vi "Sample Changer tester.vi"() -> ()   [LabVIEW 2016]
uses:
  Tester-states.ctl
  <vilib>/Analysis/NI_AALBase.lvlib
panel:
  out "Rotation Duration":u32(graph)
  out "Rotation Duration Histogram":T1(graph)
  out "End Time":timestamp
  out "Start Time":timestamp
  out "Error Histogram":T1(graph)
  out "Success rate":dbl
  in  "Trials":i32=5
  out "Sample Number":cluster{"UInt8":u8, "UInt8":u8}(graph)
  in  "Rotate minimum time":u32=5000
  out "Position error (encoder steps)":i32(graph)
  out "Encoder data":cluster{"Int32":i32, "Int32":i32}(graph)={"Int32"=515, "Int32"=0}
  out "Encoder Destination":i32
  out "Encoder Position":i32
  out "Current Sample":u8
  out "Loop Counter":i32
  in  "Encoder Radius":dbl=2.0
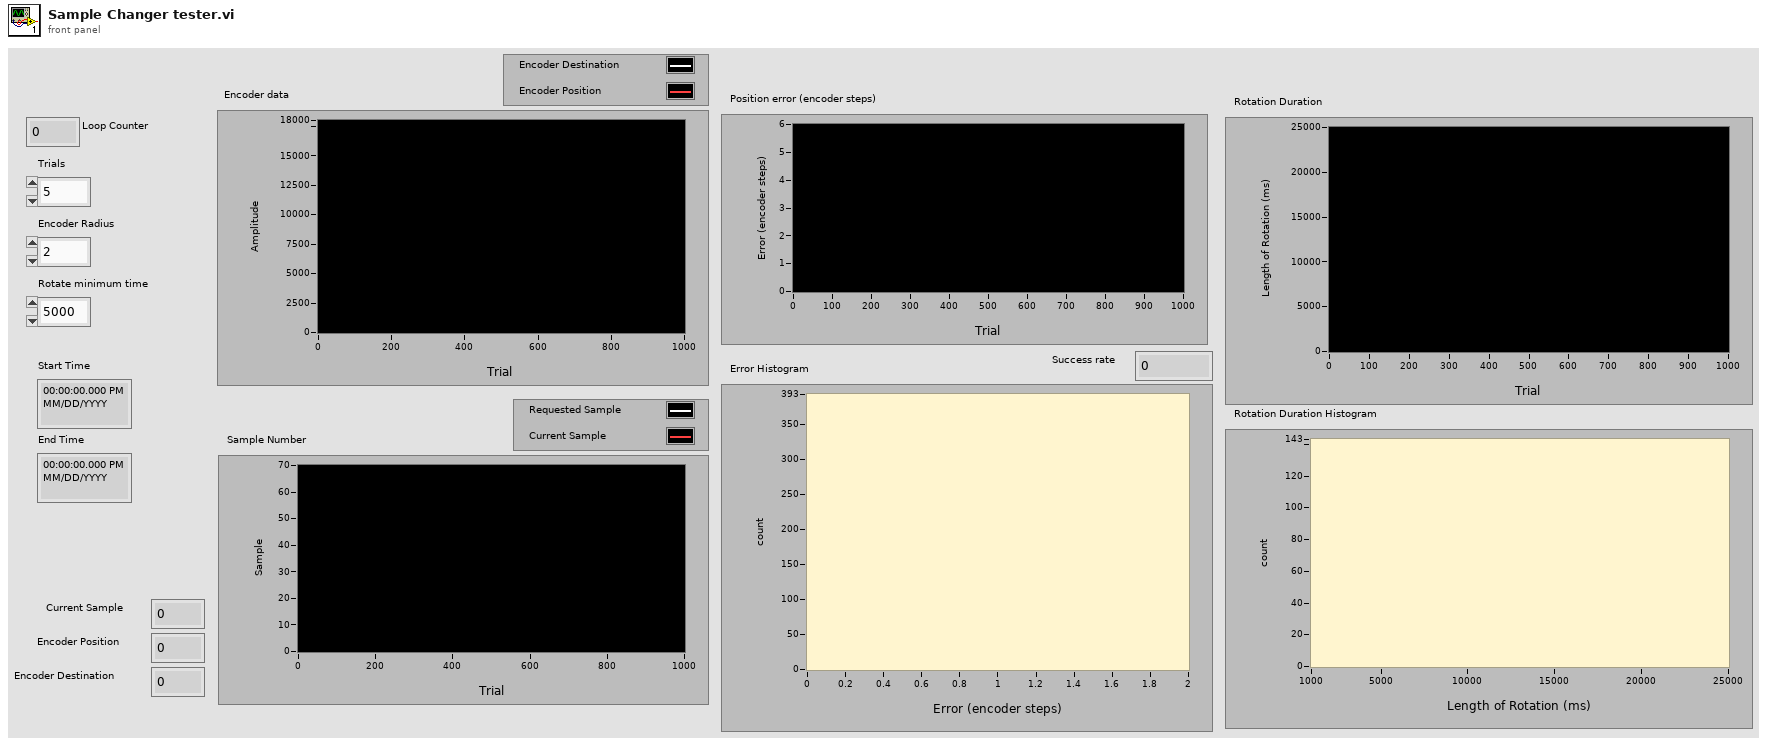
[diagram p1: front panel]
types:
  T1 = cluster{"X Values":dbl[], "Histogram: h(x)":i32[]}
  T2 = typedef "Tester-states.ctl" = enum16{"wait", "start trial", "get trial data", "test complete"}
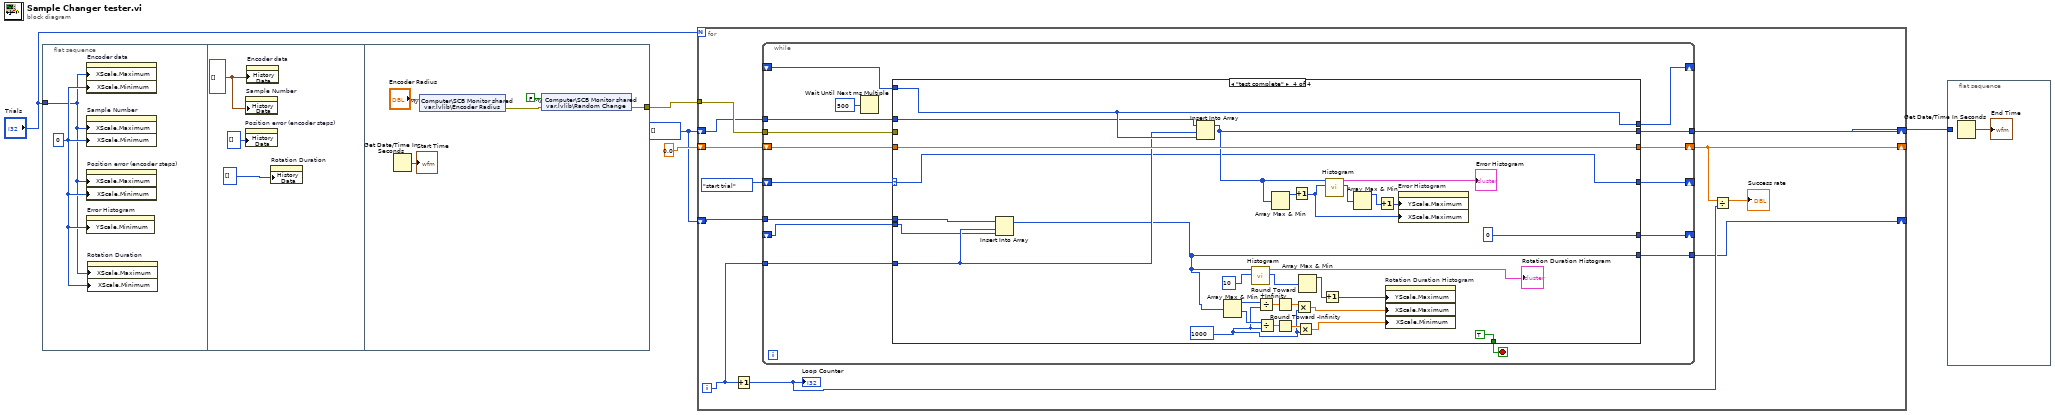
[diagram p0: block diagram]
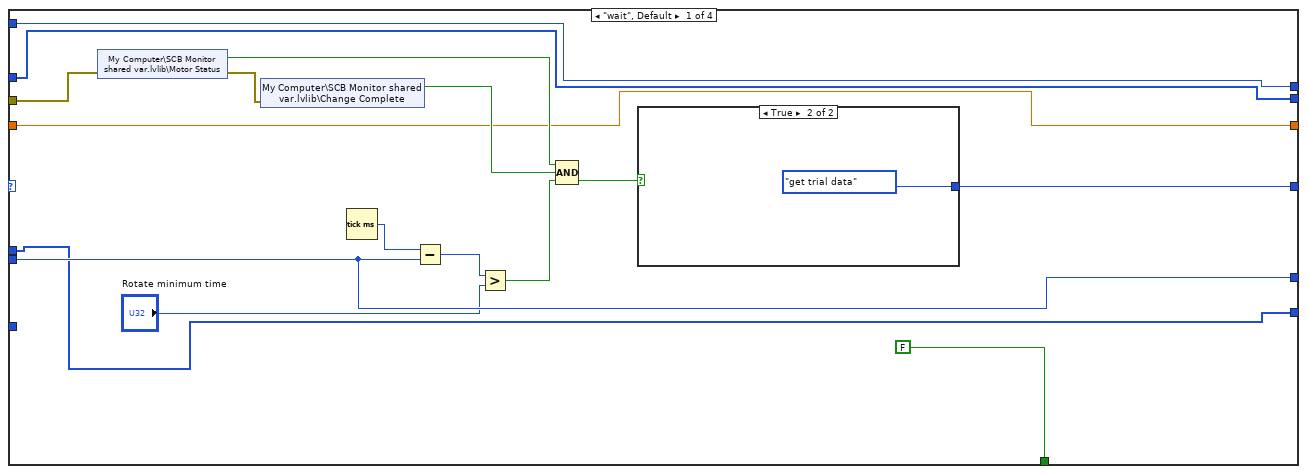
[diagram p2: hidden frame]
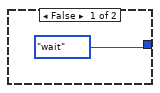
[diagram p3: hidden frame]
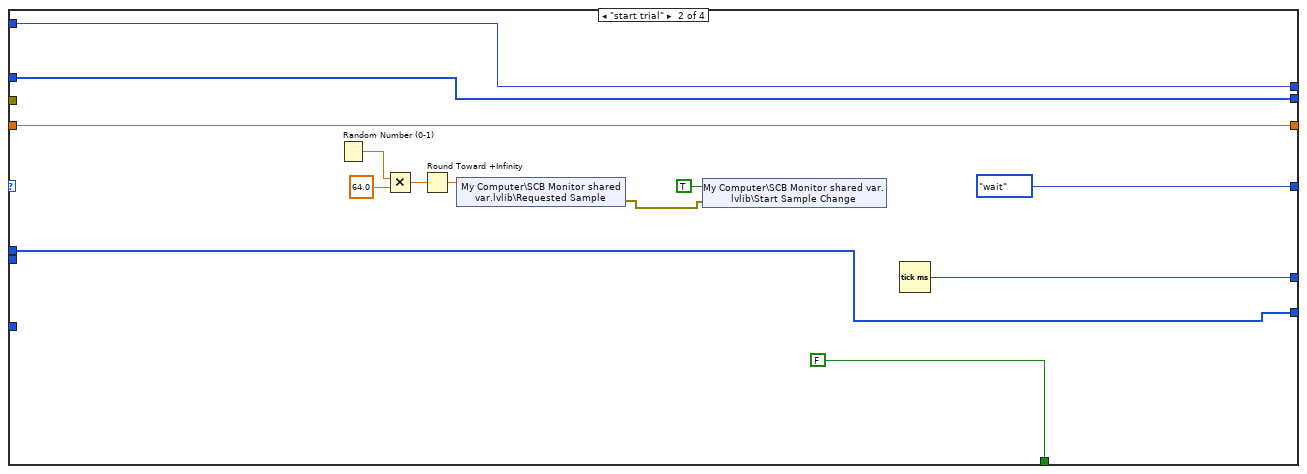
[diagram p4: hidden frame]
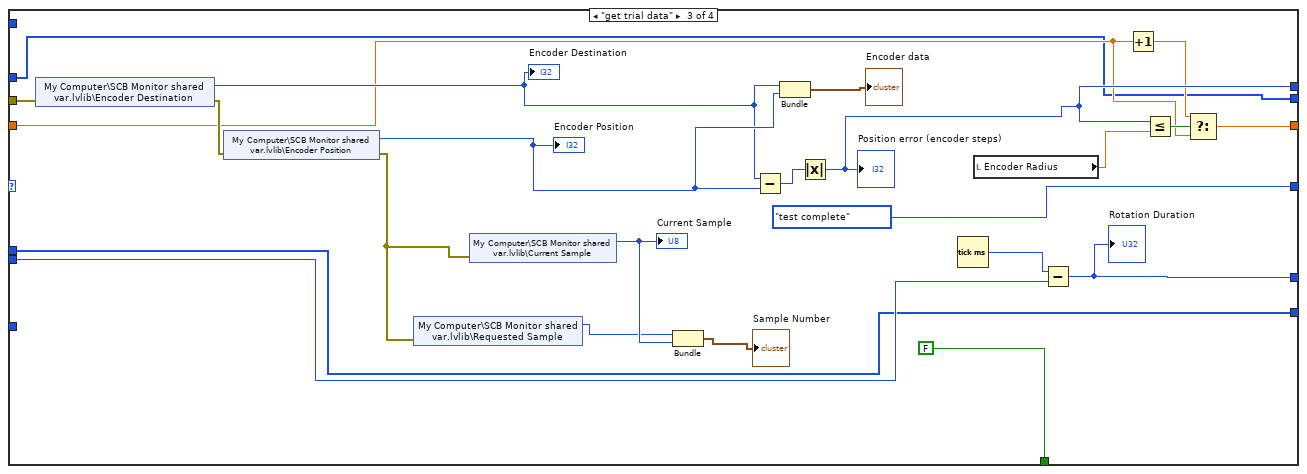
[diagram p5: hidden frame]
diagram:
  w1 = i32[] []
  n1 = flat-sequence {
    tunnel: "Trials" -> [w6]
    tunnel: [w12] -> w5
    frame #0 {
      w7 = 0 ("Trials 2")
      n2 = property on="Encoder data" class="WFChart (strict)"("XScale.Maximum"=w6, "XScale.Minimum"=w7) -> ()  [unwired: 2 in, 2 out]
      n3 = property on="Sample Number" class="WFChart (strict)"("XScale.Maximum"=w6, "XScale.Minimum"=w7) -> ()  [unwired: 2 in, 2 out]
      n4 = property on="Position error (encoder steps)" class="WFChart (strict)"("XScale.Maximum"=w6, "XScale.Minimum"=w7) -> ()  [unwired: 2 in, 2 out]
      n5 = property on="Error Histogram" class="XYGraph (strict)"("YScale.Minimum"=w7) -> ()  [unwired: 2 in, 2 out]
      n6 = property on="Rotation Duration" class="WFChart (strict)"("XScale.Maximum"=w6, "XScale.Minimum"=w7) -> ()  [unwired: 2 in, 2 out]
    }
    frame #1 {
      w9 = cluster{"Int32":i32, "Int32":i32}[] [] ("History Data")
      n7 = property on="Position error (encoder steps)" class="WFChart (strict)"("History Data"=i32[] []) -> ()  [unwired: 2 in, 2 out]
      n8 = property on="Sample Number" class="WFChart (strict)"("History Data"=w9) -> ()  [unwired: 2 in, 2 out]
      n9 = property on="Encoder data" class="WFChart (strict)"("History Data"=w9) -> ()  [unwired: 2 in, 2 out]
      n10 = property on="Rotation Duration" class="WFChart (strict)"("History Data"=i32[] []) -> ()  [unwired: 2 in, 2 out]
    }
    frame #2 {
      n11 = Get Date/Time In Seconds() -> (seconds since 1Jan1904=→"Start Time":timestamp)
      n12 = shared-variable "My Computer\\SCB Monitor shared var.lvlib\\Encoder Radius"("Encoder Radius") -> (error out=w15:errorcluster)  [unwired: 1 in]
      n13 = shared-variable "My Computer\\SCB Monitor shared var.lvlib\\Random Change"(FALSE ("Random Change"), error in=w15) -> (error out=w12:errorcluster)
    }
  }
  n14 = for {
    N: "Trials" -> [_]
    tunnel: w5 -> [w25]
    shift-right: [w21] -> _
    shift-left: 0.0 -> [w24]
    shift-right: [w19] -> w2
    shift-left: w1 -> [w18]
    shift-right: [w16] -> _
    shift-left: w1 -> [w17]
    i -> [w20]
    n15 = Increment(x=w20) -> (x+1=w22:i32)
    "Loop Counter" <- w22
    n16 = while {
      shift-right: [w40] -> _
      shift-left: Tester-states."start trial" -> [w39]
      tunnel: w25 -> [w38]
      shift-right: [w37] -> _
      shift-left: _ -> [w36]
      shift-right: [w34] -> _
      shift-left: _ -> [w35]
      shift-right: [w33] -> w21
      shift-left: w24 -> [w32]
      tunnel: w20 -> [w31]
      tunnel: [w30] -> w19
      tunnel: w18 -> [w29]
      tunnel: w17 -> [w28]
      tunnel: [w27] -> w16
      stop <- w42 stop-if-true
      n17 = Wait Until Next ms Multiple(millisecond multiple=u32 500) -> ()  [unwired: 1 out]
      n18 = case shown="\"test complete\"" w39 {
        selector: w39 -> [_ _ _ w112]
        tunnel: [FALSE FALSE FALSE TRUE] -> w42
        tunnel: [w57 Tester-states."wait" Tester-states."test complete" w112] -> w40
        tunnel: w38 -> [w49 _ w92 _]
        tunnel: [w51 w65 w74 u32 0 ("millisecond timer value")] -> w37
        tunnel: w36 -> [w51 _ w76 w114]
        tunnel: w35 -> [w46 w64 _ w124]
        tunnel: [w46 w64 w84 w124] -> w34
        tunnel: [w45 w63 w81 w125] -> w33
        tunnel: w32 -> [w45 w63 w80 w125]
        tunnel: w31 -> [_ _ _ w115]
        tunnel: [w44 w62 w78 w116] -> w30
        tunnel: w29 -> [w44 w62 w78 w123]
        tunnel: w28 -> [w43 w61 w75 w113]
        tunnel: [w43 w61 w75 w106] -> w27
        frame "wait", Default {
          n19 = shared-variable "My Computer\\SCB Monitor shared var.lvlib\\Motor Status"(error in=w49) -> (w50:bool, error out=w48:errorcluster)
          n20 = shared-variable "My Computer\\SCB Monitor shared var.lvlib\\Change Complete"(error in=w48) -> (w54:bool)  [unwired: 1 out]
          n21 = Tick Count (ms)() -> (millisecond timer value=w56:u32)
          n22 = Subtract(x=w56, y=w51) -> (x-y=w53:u32)
          n23 = Greater?(x=w53, y="Rotate minimum time") -> (0:w52:bool)
          n24 = Compound Arithmetic op=AND(w50, w54, w52) -> (w55:bool)
          n25 = case shown="True" w55 {
            tunnel: [Tester-states."wait" Tester-states."get trial data"] -> w57
            frame False {
            }
            frame True {
            }
          }
        }
        frame "start trial" {
          n26 = Random Number (0-1)() -> (number: 0 to 1=w69:dbl)
          n27 = Multiply(x=w69, y=64.0) -> (x*y=w70:dbl)
          n28 = Round Toward +Infinity(x=w70) -> (ceil(x): smallest int >= x=w67:dbl)
          n29 = shared-variable "My Computer\\SCB Monitor shared var.lvlib\\Requested Sample"(w67) -> (error out=w66:errorcluster)  [unwired: 1 in]
          n30 = shared-variable "My Computer\\SCB Monitor shared var.lvlib\\Start Sample Change"(TRUE ("Start Sample Change"), error in=w66) -> ()  [unwired: 1 out]
          n31 = Tick Count (ms)() -> (millisecond timer value=w65:u32)
        }
        frame "get trial data" {
          n32 = shared-variable "My Computer\\SCB Monitor shared var.lvlib\\Encoder Destination"(error in=w92) -> (w89:i32, error out=w91:errorcluster)
          "Encoder Destination" <- w89
          n33 = shared-variable "My Computer\\SCB Monitor shared var.lvlib\\Encoder Position"(error in=w91) -> (w90:i32, error out=w88:errorcluster)
          "Encoder Position" <- w90
          n34 = shared-variable "My Computer\\SCB Monitor shared var.lvlib\\Requested Sample"(error in=w88) -> (w85:u8)  [unwired: 1 out]
          n35 = shared-variable "My Computer\\SCB Monitor shared var.lvlib\\Current Sample"(error in=w88) -> (w86:u8)  [unwired: 1 out]
          "Current Sample" <- w86
          n36 = Bundle("UInt8"=w85, "UInt8"=w86) -> (→"Sample Number":cluster{"UInt8":u8, "UInt8":u8})  [unwired: 1 in]
          n37 = Subtract(x=w89, y=w90) -> (x-y=w94:i32)
          n38 = Bundle("Int32"=w89, "Int32"=w90) -> (→"Encoder data":cluster{"Int32":i32, "Int32":i32})  [unwired: 1 in]
          n39 = Absolute Value(x=w94) -> (abs(x)=w84:i32)
          "Position error (encoder steps)" <- w84
          n40 = Tick Count (ms)() -> (millisecond timer value=w77:u32)
          n41 = local read "Encoder Radius"() -> (w83:dbl)
          n42 = Subtract(x=w77, y=w76) -> (x-y=w74:u32)
          "Rotation Duration" <- w74
          n43 = Increment(x=w80) -> (x+1=w79:dbl)
          n44 = Less Or Equal?(x=w84, y=w83) -> (x <= y?=w82:bool)
          n45 = Select(t=w79, s=w82, f=w80) -> (s? t:f=w81:dbl)
        }
        frame "test complete" {
          w99 = 1000 ("y")
          n46 = Insert Into Array(array=w113, index=w115, new element=w114) -> (w106:i32[])
          n47 = Insert Into Array(array=w123, index=w115, new element=w124) -> (w116:i32[])
          n48 = Array Max & Min(array=w106) -> (max value=w105:i32, min value=w104:i32)  [unwired: 2 out]
          n49 = call <vilib>:"Histogram.vi"("intervals"=10, "X"=w106) -> ("Histogram: h(x)"=w108:i32[], "Histogram Graph"=→"Rotation Duration Histogram":T1)  [unwired: 6 in, 2 out]
          n50 = Divide(x=w105, y=w99) -> (x/y=w102:dbl)
          n51 = Divide(x=w104, y=w99) -> (x/y=w103:dbl)
          n52 = Array Max & Min(array=w116) -> (max value=w122:i32)  [unwired: 3 out]
          n53 = Round Toward +Infinity(x=w102) -> (ceil(x): smallest int >= x=w101:dbl)
          n54 = Round Toward -Infinity(1:w103) -> (0:w100:dbl)
          n55 = Increment(x=w122) -> (x+1=w117:i32)
          n56 = Multiply(x=w101, y=w99) -> (x*y=w98:dbl)
          n57 = Multiply(x=w100, y=w99) -> (x*y=w97:dbl)
          n58 = Array Max & Min(array=w108) -> (max value=w109:i32)  [unwired: 3 out]
          n59 = Increment(x=w109) -> (x+1=w107:i32)
          n60 = call <vilib>:"Histogram.vi"("intervals"=w117, "X"=w116) -> ("Histogram: h(x)"=w120:i32[], "Histogram Graph"=→"Error Histogram":T1)  [unwired: 6 in, 2 out]
          n61 = Array Max & Min(array=w120) -> (max value=w119:i32)  [unwired: 3 out]
          n62 = Increment(x=w119) -> (x+1=w118:i32)
          n63 = property on="Rotation Duration Histogram" class="XYGraph (strict)"("YScale.Maximum"=w107, "XScale.Maximum"=w98, "XScale.Minimum"=w97) -> ()  [unwired: 2 in, 2 out]
          n64 = property on="Error Histogram" class="XYGraph (strict)"("YScale.Maximum"=w118, "XScale.Maximum"=w117) -> ()  [unwired: 2 in, 2 out]
        }
      }
    }
    n65 = Divide(x=w21, y=w22) -> (x/y=→"Success rate":dbl)
  }
  n66 = flat-sequence {
    tunnel: w2 -> [_]
    frame #0 {
      n67 = Get Date/Time In Seconds() -> (seconds since 1Jan1904=→"End Time":timestamp)
    }
  }
